vi "Make Hardware Connect Calls.vi"(8 "error in (no error)":errorcluster, 10 "CD In Buf":dbl[](array[numeric]), 11 "Engine Run Time Data in":T1) -> (0 "error out":errorcluster, 3 "Engine Run Time Data out":T1)   [LabVIEW 2017, in "NI 272x Resistive Simulation Custom Device Engine.lvlib"]
uses:
  NI 272x Resistive Simulation Custom Device Engine.lvlib
  Controls/Engine Run Time Data.ctl
  Controls/Compiled Engine Data.ctl
  Controls/Compiled HW Channel.ctl
  Controls/Channel Mode.ctl
  <instrlib>/ni272xReferenceVIs/ni272xReferenceVIs.llb/ni272x Callendar-Van Dusen RTD Parameters.ctl
  Controls/Compiled Connect Channel.ctl
  <instrlib>/ni272xReferenceVIs/ni272xReferenceVIs.llb/ni272x Reference.ctl
  <instrlib>/ni272xReferenceVIs/ni272xReferenceVIs.llb/ni272x Connect 2Chan.vi
  <instrlib>/ni272xReferenceVIs/ni272xReferenceVIs.llb/ni272x Disconnect 2Chan.vi
  NI 272x Resistive Simulation Custom Device Shared.lvlib
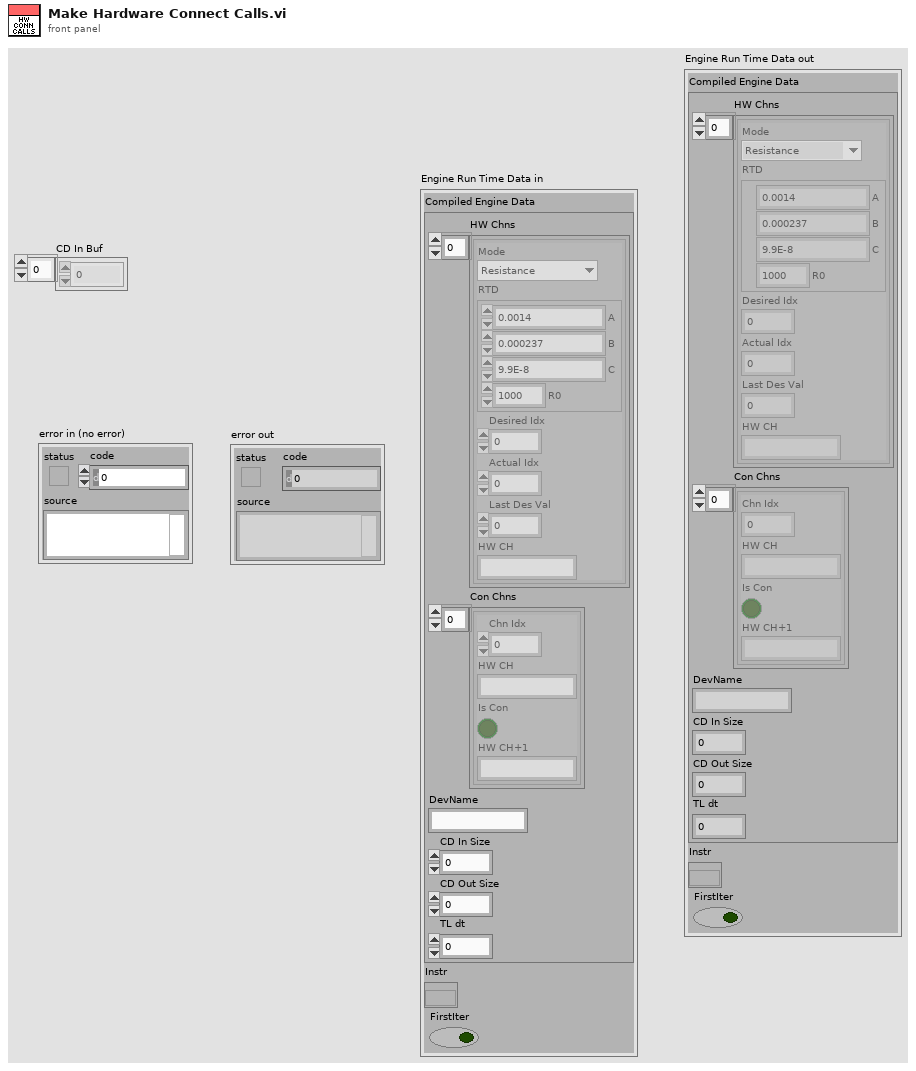
[diagram p1: front panel]
types:
  T1 = typedef "NI 272x Resistive Simulation Custom Device Engine.lvlib/Engine Run Time Data.ctl" = cluster{"Compiled Engine Data":T2, "Instr":T7, "FirstIter":bool}
  T2 = typedef "NI 272x Resistive Simulation Custom Device Shared.lvlib/Compiled Engine Data.ctl" = cluster{"HW Chns":T3[], "Con Chns":T6[], "DevName":string, "CD In Size":i32, "CD Out Size":i32, "TL dt":i64}
  T3 = typedef "NI 272x Resistive Simulation Custom Device Shared.lvlib/Compiled HW Channel.ctl" = cluster{"Mode":T4, "RTD":T5, "Desired Idx":i32, "Actual Idx":i32, "Last Des Val":dbl, "HW CH":string}
  T4 = typedef "NI 272x Resistive Simulation Custom Device Shared.lvlib/Channel Mode.ctl" = enum16{"Resistance", "RTD Temperature"}
  T5 = typedef "ni272x Callendar-Van Dusen RTD Parameters.ctl" = cluster{"A":dbl, "B":dbl, "C":dbl, "R0":dbl}
  T6 = typedef "NI 272x Resistive Simulation Custom Device Shared.lvlib/Compiled Connect Channel.ctl" = cluster{"Chn Idx":i32, "HW CH":string, "Is Con":bool, "HW CH+1":string}
  T7 = typedef "ni272x Reference.ctl" = refnum<k20>
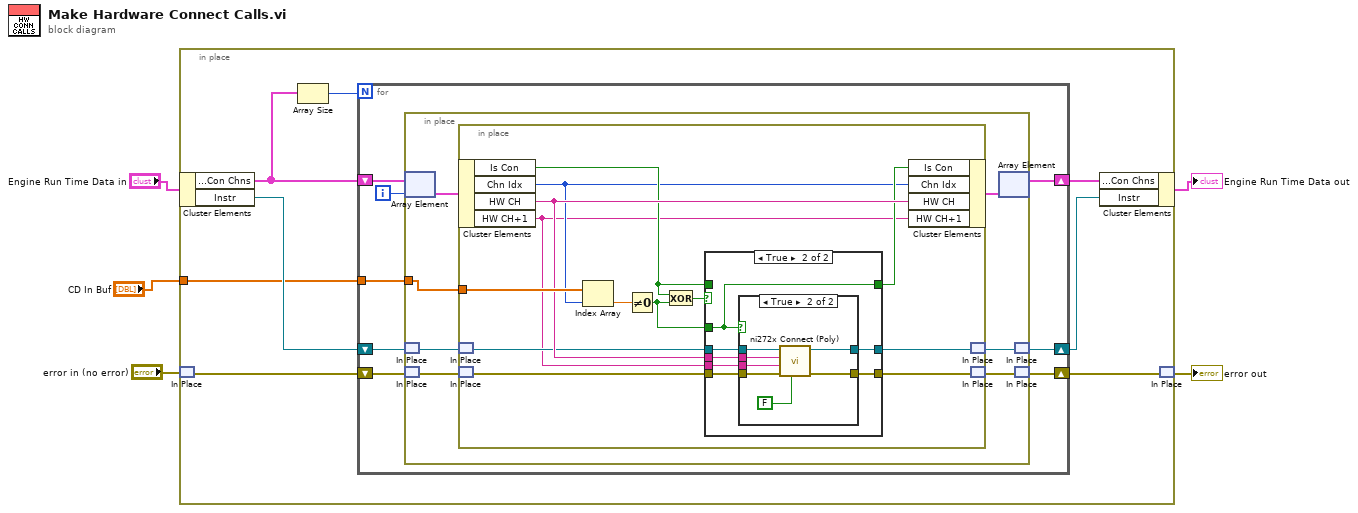
[diagram p0: block diagram]
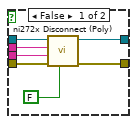
[diagram p3: hidden frame]
diagram:
  n1 = in-place {
    in-place-border: "CD In Buf" -> [w6]
    n2 = in-place-cluster #1("Engine Run Time Data in") -> ("Compiled Engine Data.Con Chns"=w10:T6[], "Instr"=w13:T7)
    n3 = in-place-match #2("error in (no error)") -> (w12:errorcluster)
    n4 = Array Size(array=w10) -> (size(s)=w11:i32)
    n5 = for {
      N: w11 -> [_]
      shift-right: [w16] -> w8
      shift-left: w13 -> [w17]
      shift-right: [w18] -> w7
      shift-left: w12 -> [w19]
      shift-right: [w15] -> w9
      shift-left: w10 -> [w21]
      tunnel: w6 -> [w14]
      i -> [w20]
      n6 = in-place {
        in-place-border: w14 -> [w22]
        n7 = in-place-array #3(w21, w20) -> (w28:T6)
        n8 = in-place-match #4(w17) -> (w24:T7)
        n9 = in-place-match #5(w19) -> (w27:errorcluster)
        n10 = in-place {
          in-place-border: w22 -> [w41]
          n11 = in-place-cluster #6(w28) -> ("Is Con"=w31:bool, "Chn Idx"=w30:i32, "HW CH"=w40:string, "HW CH+1"=w29:string)
          n12 = in-place-match #7(w24) -> (w37:T7)
          n13 = in-place-match #8(w27) -> (w39:errorcluster)
          n14 = Index Array(array=w41, index=w30) -> (element=w35:dbl)
          n15 = Not Equal To 0?(x=w35) -> (x != 0?=w33:bool)
          n16 = Exclusive Or(1:w33, 2:w31) -> (0:w34:bool)
          n17 = case shown="True" w34 {
            tunnel: w40 -> [_ w49]
            tunnel: w39 -> [w44 w51]
            tunnel: w37 -> [w43 w50]
            tunnel: [w44 w48] -> w38
            tunnel: [w43 w47] -> w36
            tunnel: w29 -> [_ w46]
            tunnel: w33 -> [_ w45]
            tunnel: [w42 w45] -> w32
            tunnel: w31 -> [w42 _]
            frame False {
            }
            frame True {
              n18 = case shown="True" w45 {
                tunnel: w51 -> [w58 w65]
                tunnel: w50 -> [w57 w62]
                tunnel: w49 -> [w56 w61]
                tunnel: [w52 w64] -> w48
                tunnel: [w53 w63] -> w47
                tunnel: w46 -> [w55 w60]
                frame False {
                  n19 = call-poly <instrlib>:"ni272x Disconnect (Poly).vi"("wait for settling (T)"=FALSE, "error in (no error)"=w58, "resistor channel N+1"=w55, "resistor channel N"=w56, "instrument handle"=w57) -> ("error out"=w52:errorcluster, "instrument handle out"=w53:T7)  [unwired: 5 out]
                }
                frame True {
                  n20 = call-poly <instrlib>:"ni272x Connect (Poly).vi"("wait for settling (T)"=FALSE, "error in (no error)"=w65, "resistor channel N+1"=w60, "resistor channel N"=w61, "instrument handle"=w62) -> ("error out"=w64:errorcluster, "instrument handle out"=w63:T7)  [unwired: 5 out]
                }
              }
            }
          }
          n21 = in-place-cluster #6("Is Con"=w32, "Chn Idx"=w30, "HW CH"=w40, "HW CH+1"=w29) -> (w25:T6)
          n22 = in-place-match #7(w36) -> (w23:T7)
          n23 = in-place-match #8(w38) -> (w26:errorcluster)
        }
        n24 = in-place-array #3(w25) -> (w15:T6[])  [unwired: 1 out]
        n25 = in-place-match #4(w23) -> (w16:T7)
        n26 = in-place-match #5(w26) -> (w18:errorcluster)
      }
    }
    n27 = in-place-cluster #1("Compiled Engine Data.Con Chns"=w9, "Instr"=w8) -> (→"Engine Run Time Data out":T1)
    n28 = in-place-match #2(w7) -> (→"error out":errorcluster)
  }
